vi "Configure Probability.vi"(8 "error in (no error)":errorcluster, 9 "Number Of Histogram Bins (0: eb64)":i32(ring) items=["eb64", "eb128", "eb256", "eb512", "eb1024"], 10 "Calculate Probability (T: Enable)":bool=TRUE, 11 "VISA resource name":refnum<visa-resource-name>) -> (0 "error out":errorcluster, 3 "VISA resource name out":refnum<visa-resource-name>)   [LabVIEW 2014, in "Stanford Research SR1.lvlib"]
doc: "Configures the attributes for the Probability."
uses:
  Stanford Research SR1.lvlib
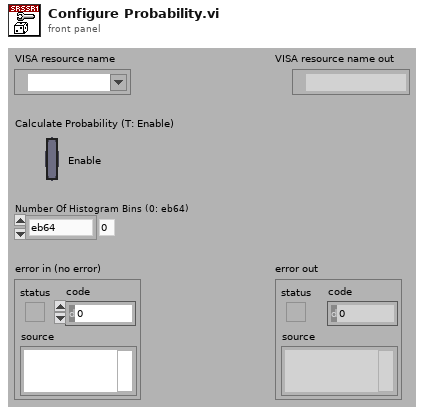
[diagram p1: front panel]
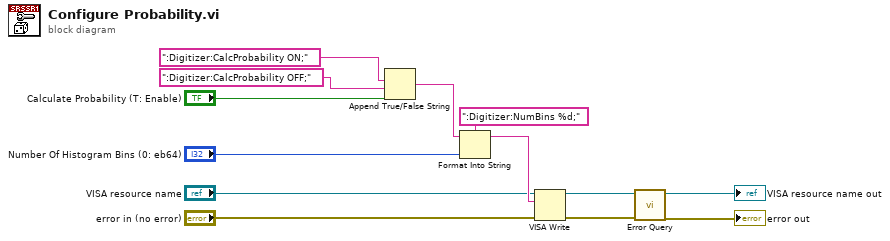
[diagram p0: block diagram]
diagram:
  n1 = Append True/False String(1:"Calculate Probability (T: Enable)", 2:":Digitizer:CalcProbability OFF;", 3:":Digitizer:CalcProbability ON;") -> (0:w10:string)  [unwired: 1 in]
  n2 = Format Into String(format string=":Digitizer:NumBins %d;", initial string=w10, "Number Of Histogram Bins (0: eb64)") -> (resulting string=w7:string)  [unwired: 1 in, 1 out]
  n3 = VISA Write(VISA resource name="VISA resource name", write buffer=w7, error in (no error)="error in (no error)") -> (VISA resource name out=w4:refnum<visa-resource-name>, error out=w3:errorcluster)  [unwired: 1 out]
  n4 = call "Error Query.vi"("error in (no error)"=w3, "VISA resource name"=w4) -> ("error out"=→"error out":errorcluster, "VISA resource name out"=→"VISA resource name out":refnum<visa-resource-name>)  [unwired: 6 in, 2 out]
